vi "PH_SHS_Analysis_Statistician.handle Data.vi"(6 "New SHS Analyzer Dataset":T1 {"State" items=["no info", "off/false/out", "on/true/in", "Failure", "Alarm", "Status 1", "Status 2", "Status 3"]; "Zernicke Coefficients"."2nd Spherical" scale=-2.0..2.0 scale format="%.2f"; "Zernicke Coefficients"."2nd Coma y" scale=-2.0..2.0 scale format="%.2f"; "Zernicke Coefficients"."2nd Coma x" scale=-2.0..2.0 scale format="%.2f"; "Zernicke Coefficients"."2nd Astig 45°" scale=-2.0..2.0 scale format="%.2f"; "Zernicke Coefficients"."2nd Astig 0°" scale=-2.0..2.0 scale format="%.2f"; "Zernicke Coefficients"."Trefoil 30°" scale=-2.0..2.0 scale format="%.2f"; "Zernicke Coefficients"."Trefoil 0°" scale=-2.0..2.0 scale format="%.2f"; "Zernicke Coefficients"."Spherical" scale=-2.0..2.0 scale format="%.2f"; "Zernicke Coefficients"."Coma y" scale=-2.0..2.0 scale format="%.2f"; "Zernicke Coefficients"."Coma x" scale=-2.0..2.0 scale format="%.2f"; "Zernicke Coefficients"."Astig 45°" scale=-2.0..2.0 scale format="%.2f"; "Zernicke Coefficients"."Astig 0°" scale=-2.0..2.0 scale format="%.2f"; "Zernicke Coefficients"."Defocus" scale=-2.0..2.0 scale format="%.2f"; "Zernicke Coefficients"."Tilt y" scale=-2.0..2.0 scale format="%.2f"; "Zernicke Coefficients"."Tilt x" scale=-2.0..2.0 scale format="%.2f"}, 7 "Dataarray Size in":i32, 8 "Data in":T1[](array[typedef]) {"State" items=["no info", "off/false/out", "on/true/in", "Failure", "Alarm", "Status 1", "Status 2", "Status 3"]; "Zernicke Coefficients"."2nd Spherical" scale=-2.0..2.0 scale format="%.2f"; "Zernicke Coefficients"."2nd Coma y" scale=-2.0..2.0 scale format="%.2f"; "Zernicke Coefficients"."2nd Coma x" scale=-2.0..2.0 scale format="%.2f"; "Zernicke Coefficients"."2nd Astig 45°" scale=-2.0..2.0 scale format="%.2f"; "Zernicke Coefficients"."2nd Astig 0°" scale=-2.0..2.0 scale format="%.2f"; "Zernicke Coefficients"."Trefoil 30°" scale=-2.0..2.0 scale format="%.2f"; "Zernicke Coefficients"."Trefoil 0°" scale=-2.0..2.0 scale format="%.2f"; "Zernicke Coefficients"."Spherical" scale=-2.0..2.0 scale format="%.2f"; "Zernicke Coefficients"."Coma y" scale=-2.0..2.0 scale format="%.2f"; "Zernicke Coefficients"."Coma x" scale=-2.0..2.0 scale format="%.2f"; "Zernicke Coefficients"."Astig 45°" scale=-2.0..2.0 scale format="%.2f"; "Zernicke Coefficients"."Astig 0°" scale=-2.0..2.0 scale format="%.2f"; "Zernicke Coefficients"."Defocus" scale=-2.0..2.0 scale format="%.2f"; "Zernicke Coefficients"."Tilt y" scale=-2.0..2.0 scale format="%.2f"; "Zernicke Coefficients"."Tilt x" scale=-2.0..2.0 scale format="%.2f"}, 9 "Datasets strored in":i32) -> (1 "Dataarray Size out":i32, 2 "Data out":T1[](array[typedef]) {"State" items=["no info", "off/false/out", "on/true/in", "Failure", "Alarm", "Status 1", "Status 2", "Status 3"]; "Zernicke Coefficients"."2nd Spherical" scale=-2.0..2.0 scale format="%.2f"; "Zernicke Coefficients"."2nd Coma y" scale=-2.0..2.0 scale format="%.2f"; "Zernicke Coefficients"."2nd Coma x" scale=-2.0..2.0 scale format="%.2f"; "Zernicke Coefficients"."2nd Astig 45°" scale=-2.0..2.0 scale format="%.2f"; "Zernicke Coefficients"."2nd Astig 0°" scale=-2.0..2.0 scale format="%.2f"; "Zernicke Coefficients"."Trefoil 30°" scale=-2.0..2.0 scale format="%.2f"; "Zernicke Coefficients"."Trefoil 0°" scale=-2.0..2.0 scale format="%.2f"; "Zernicke Coefficients"."Spherical" scale=-2.0..2.0 scale format="%.2f"; "Zernicke Coefficients"."Coma y" scale=-2.0..2.0 scale format="%.2f"; "Zernicke Coefficients"."Coma x" scale=-2.0..2.0 scale format="%.2f"; "Zernicke Coefficients"."Astig 45°" scale=-2.0..2.0 scale format="%.2f"; "Zernicke Coefficients"."Astig 0°" scale=-2.0..2.0 scale format="%.2f"; "Zernicke Coefficients"."Defocus" scale=-2.0..2.0 scale format="%.2f"; "Zernicke Coefficients"."Tilt y" scale=-2.0..2.0 scale format="%.2f"; "Zernicke Coefficients"."Tilt x" scale=-2.0..2.0 scale format="%.2f"}, 3 "Datasets strored out":i32)   [LabVIEW 2014, in "PH_SHS_Analysis_Statistician.lvlib"]
doc: "This VI handles the array made out of new dataset coming in: It creates an array of 3600 enries (values NaN) and replaces them peu a peu by the new incoming dataset. If the array is full, additional 3600 NaN-entries are added and so on ..."
uses:
  PH_SHS_Analysis_Statistician.lvlib
  PH_SHS_Analysis/PH_SHS_Analysis.Zernike Dataset.ctl
  PH_Basics/PH_StatusHandler/PH_StatusHandler.Status.ctl
  PH_SHS_Analysis/PH_SHS_Analysis.Zernike Coefficients.ctl
  PH_SHS_Analysis/PH_SHS_Analysis.lvlib
  PH_Basics/PH_StatusHandler/PH_StatusHandler.lvlib
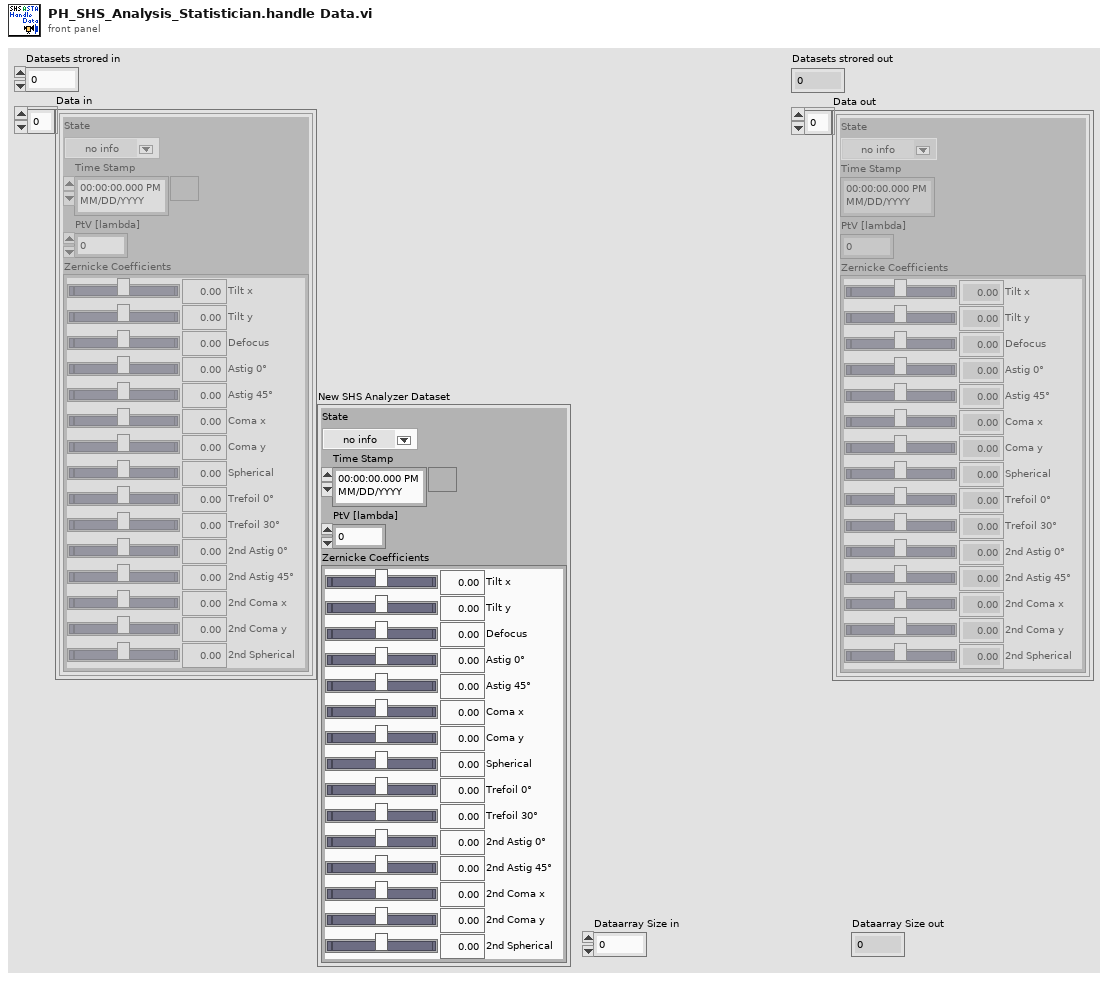
[diagram p1: front panel]
types:
  T1 = typedef "PH_SHS_Analysis.lvlib/PH_SHS_Analysis.Zernike Dataset.ctl" = cluster{"State":T2, "Time Stamp":timestamp, "PtV [lambda]":dbl, "Zernicke Coefficients":T3}
  T2 = typedef "PH_StatusHandler.lvlib/PH_StatusHandler.Status.ctl" = i16
  T3 = typedef "PH_SHS_Analysis.lvlib/PH_SHS_Analysis.Zernike Coefficients.ctl" = cluster{"Tilt x":dbl, "Tilt y":dbl, "Defocus":dbl, "Astig 0°":dbl, "Astig 45°":dbl, "Coma x":dbl, "Coma y":dbl, "Spherical":dbl, "Trefoil 0°":dbl, "Trefoil 30°":dbl, "2nd Astig 0°":dbl, "2nd Astig 45°":dbl, "2nd Coma x":dbl, "2nd Coma y":dbl, "2nd Spherical":dbl}
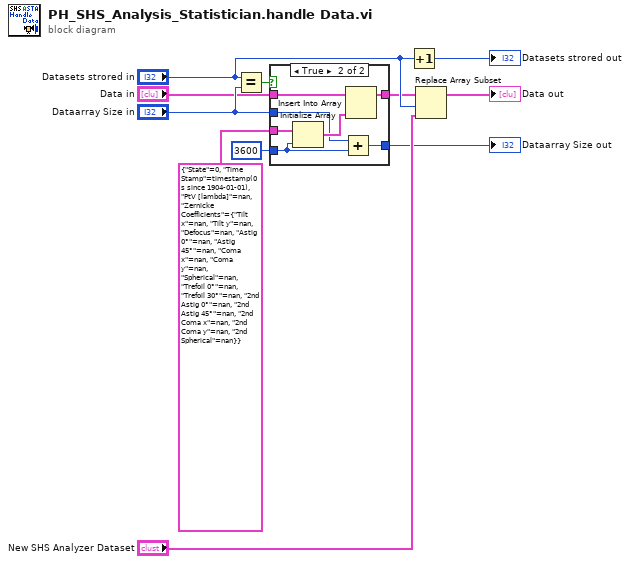
[diagram p0: block diagram]
diagram:
  n1 = Equal?(x="Datasets strored in", y="Dataarray Size in") -> (x = y?=w11:bool)
  n2 = case shown="True" w11 {
    tunnel: "Data in" -> [w13 w20]
    tunnel: [w13 w19] -> w8
    tunnel: "Dataarray Size in" -> [w12 w17]
    tunnel: [w12 w16] -> w4
    tunnel: T1 {"State"=0, "Time Stamp"=timestamp(0 s since 1904-01-01), "PtV [lambda]"=nan, "Zernicke Coefficients"={"Tilt x"=nan, "Tilt y"=nan, "Defocus"=nan, "Astig 0°"=nan, "Astig 45°"=nan, "Coma x"=nan, "Coma y"=nan, "Spherical"=nan, "Trefoil 0°"=nan, "Trefoil 30°"=nan, "2nd Astig 0°"=nan, "2nd Astig 45°"=nan, "2nd Coma x"=nan, "2nd Coma y"=nan, "2nd Spherical"=nan}} ("New SHS Analyzer Dataset 2") -> [_ w15]
    tunnel: 3600 ("dimension size") -> [_ w14]
    frame False {
    }
    frame True {
      n3 = Initialize Array(w15, w14) -> (w18:T1[])
      n4 = Add(x=w17, y=w14) -> (x+y=w16:i32)
      n5 = Insert Into Array(array=w20, new element=w18) -> (w19:T1[])  [unwired: 1 in]
    }
  }
  "Dataarray Size out" <- w4
  n6 = Increment(x="Datasets strored in") -> (x+1=→"Datasets strored out":i32)
  n7 = Replace Array Subset(array=w8, new element="New SHS Analyzer Dataset", index="Datasets strored in") -> (→"Data out":T1[])
